vi "Draw Cross(45 Deg).vi"(6 "Draw Para":T1={"color(black)"=0, "pen"={"Width"=1, "Style"=enum."Solid"}}, 8 "错误输入":errorcluster, 9 "radius":i16=4 caption="半径", 10 "Center":T2, 11 "Pic in":picture) -> (0 "错误输出":errorcluster, 3 "Pic out":picture)   [LabVIEW 2011, in "Basic Shape.lvlib"]
uses:
  Basic Shape.lvlib
  Point Custom Control.ctl
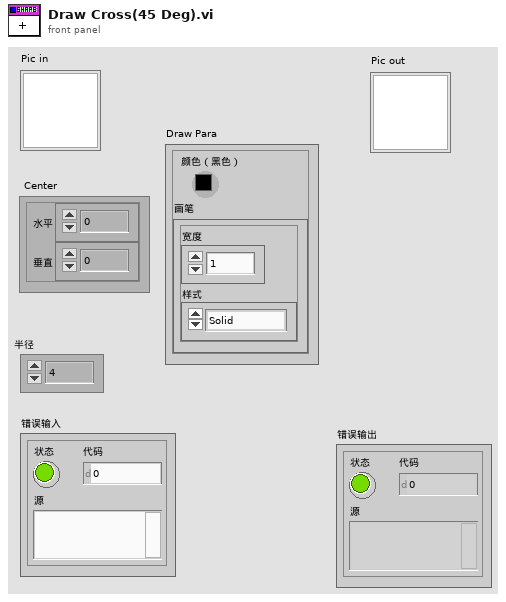
[diagram p1: front panel]
types:
  T1 = cluster{"color(black)":u32, "pen":cluster{"Width":u16, "Style":enum32{"Solid", "Dash", "Dot", "DashDot", "DashDotDot"}}}
  T2 = typedef "Basic Shape.lvlib/Point Custom Control.ctl" = cluster{"horizontal":i16, "vertical":i16}
  T3 = cluster{"Width":u16, "Style":enum32{"Solid", "Dash", "Dot", "DashDot", "DashDotDot"}}
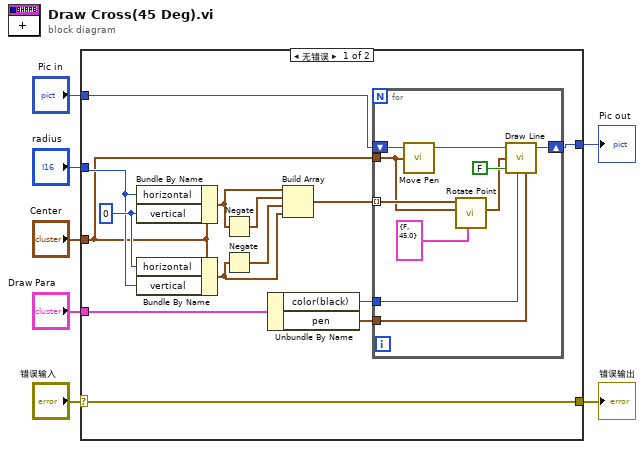
[diagram p0: block diagram]
diagram:
  n1 = case shown="无错误" "错误输入" {
    selector: "错误输入" -> [w21 w33]
    tunnel: [w21 w33] -> w6
    tunnel: "Pic in" -> [w17 w32]
    tunnel: "Center" -> [w14 _]
    tunnel: "Draw Para" -> [w20 _]
    tunnel: "radius" -> [w15 _]
    tunnel: [w8 w32] -> w1
    frame No Error {
      w16 = i16 0 ("vertical")
      n2 = Bundle By Name(cluster=w14, "horizontal"=w15, "vertical"=w16) -> (w13:T2)
      n3 = Bundle By Name(cluster=w14, "horizontal"=w16, "vertical"=w15) -> (w10:T2)
      n4 = Negate(x=w13) -> (-x=w12:T2)
      n5 = Negate(x=w10) -> (-x=w11:T2)
      n6 = Unbundle By Name(w20) -> ("color(black)"=w19:u32, "pen"=w18:T3)
      n7 = Build Array(w13, w12, w11, w10) -> (w9:T2[])
      n8 = for {
        tunnel: w19 -> [w31]
        tunnel: w18 -> [w30]
        tunnel: w14 -> [w24]
        shift-right: [w26] -> w8
        shift-left: w17 -> [w29]
        tunnel: w9 -> [w25] mode=indexing
        n9 = call <vilib>:"Move Pen.vi"("new position"=w24, "picture"=w29) -> ("new picture"=w28:picture)  [unwired: 3 in]
        n10 = call "Rotate Point.vi"("Para"=cluster{"Absolute?":bool, "Angle":dbl} {"Absolute?"=FALSE, "Angle"=45.0}, "Center"=w24, "Input Point"=w25) -> ("Rotated Relative Point"=w23:T2)  [unwired: 6 in, 2 out]
        n11 = call <vilib>:"Draw Line.vi"("picture"=w28, "end point"=w23, "absolute coordinates?(T)"=FALSE, "color(black)"=w31, "pen"=w30) -> ("new picture"=w26:picture)  [unwired: 4 in]
      }
    }
    frame Error {
    }
  }
  "错误输出" <- w6
  "Pic out" <- w1
